vi "Server Main.vi"() -> ()   [LabVIEW 2024]
doc: "This VI is the main VI of the server."
uses:
  Controls/Server/Server - Data.ctl
  Support/Shared/Message Queue/Server Message Queues.ctl
  Support/Shared/Message Queue/Message Cluster.ctl
  Controls/Server/Server Status.ctl
  Error Handlers/Error Message.ctl
  Controls/Server/Historical Log.ctl
  Globals/Global - Server.vi
  Support/Shared/Message Queue.lvlib
  Support/Shared/User Event - Stop.lvlib
panel:
  in  "Exit":bool
  out "Status Log":i32(listbox)=-1
  in  "Administrator Console":bool
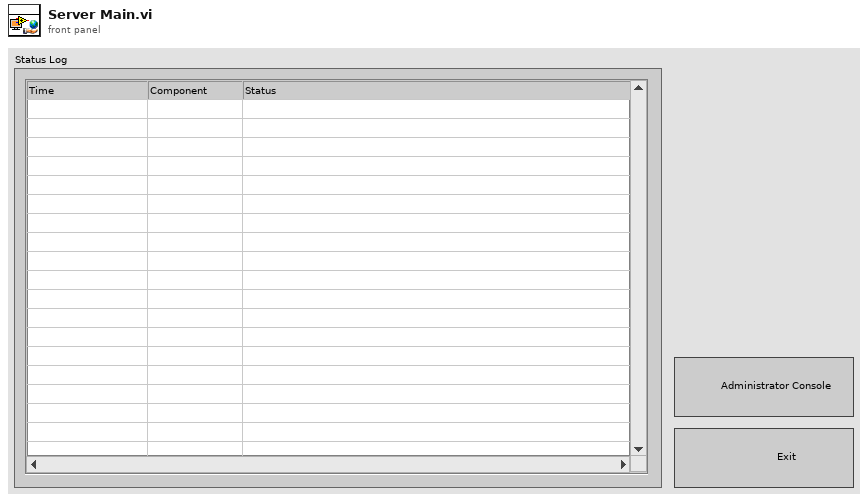
[diagram p1: front panel]
types:
  T1 = typedef "Server Status.ctl" = enum16{"Started", "Initialized", "Stopping", "Stopped"}
  T2 = typedef "Server - Data.ctl" = cluster{"UI Message Loop Initialized?":bool, "Shared Variable Management Loop Initialized?":bool, "Archive Loop Initialized?":bool, "Shared Variable Management Loop Stopped?":bool, "Archive Loop Stopped?":bool, "Administrator Console VI Reference":refnum<vi>, "Server Stop Handler":refnum<user-event>, "Server Message Queues":T3, "Server Status":T1, "Status Log Control":refnum<vi>}
  T3 = typedef "Message Queue.lvlib/Server Message Queues.ctl" = cluster{"UI":refnum<queue>, "Archive":refnum<queue>, "Shared Variable Management":refnum<queue>, "Administrator Console":refnum<queue>}
  T4 = typedef "Error Message.ctl" = cluster{"Error":errorcluster, "Component":string}
  T5 = typedef "Historical Log.ctl" = cluster{"Time":timestamp, "Component":string, "Status":string}
  T6 = typedef "System Configuration.ctl" = cluster{"Name":string, "Description":string, "Logging Computer Name":string, "Logging Database Name":string, "Logging Database Path":path, "Archive Computer Name":string, "Archive Database Name":string, "Archive Database Path":path, "Lifespan (days)":u32, "Archive Enabled":bool, "Archive Interval (hours)":u32, "Subsystems":T7[]}
  T7 = typedef "Subsystem Configuration.ctl" = cluster{"Name":string, "Root URL":refnum<k21>}
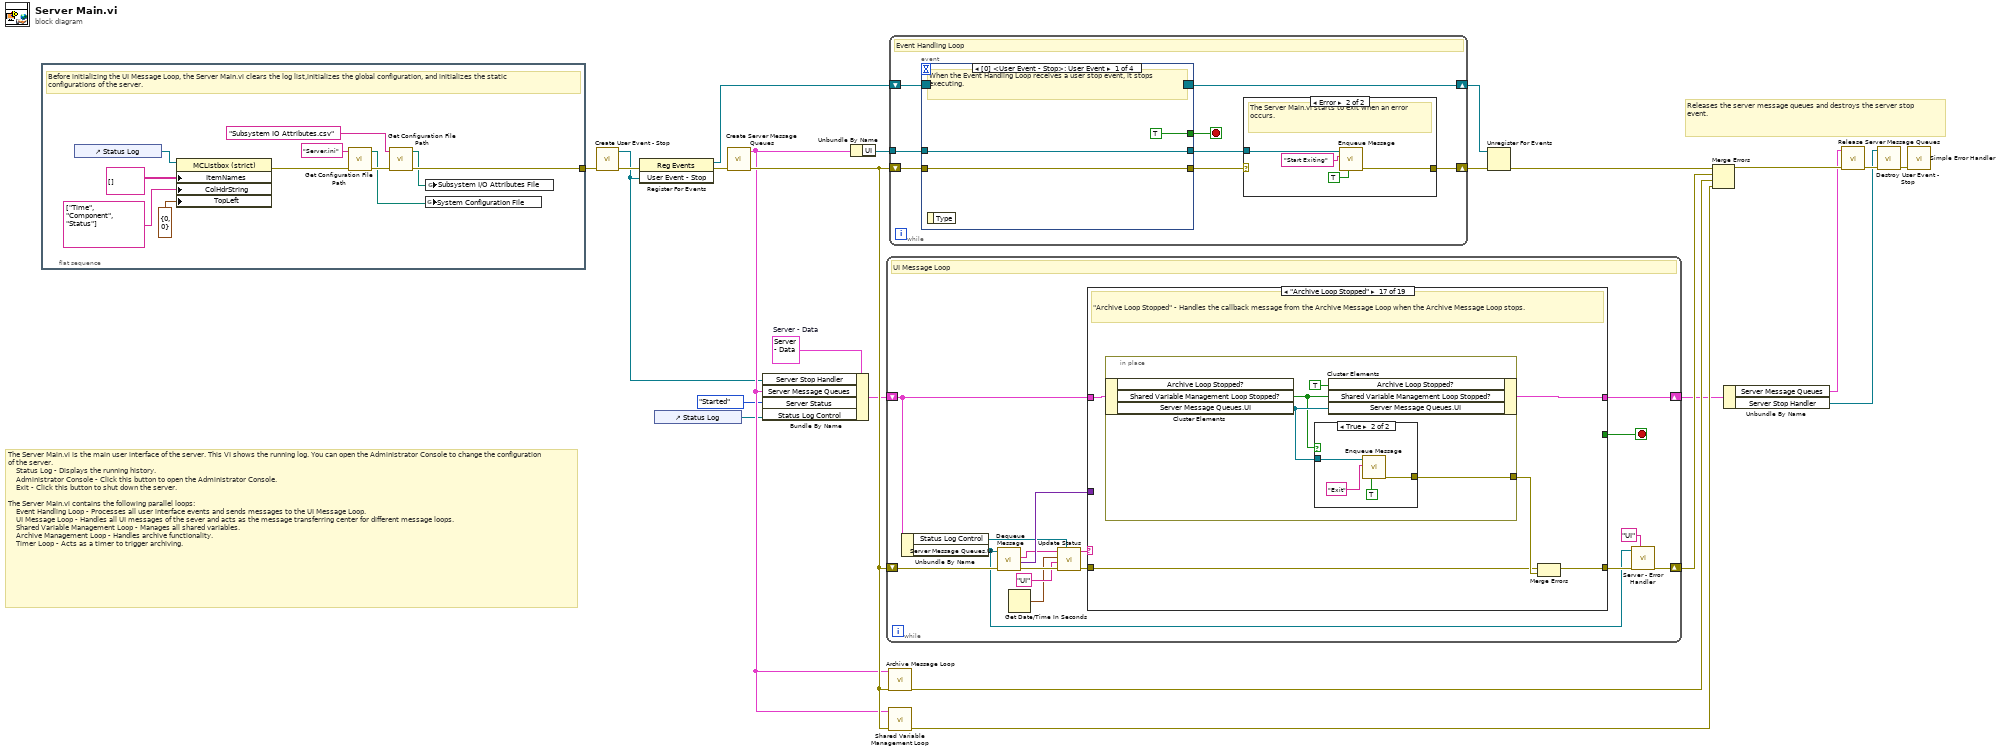
[diagram p0: block diagram]
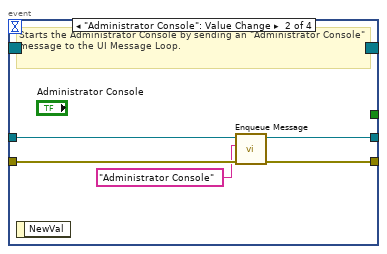
[diagram p3: hidden frame]
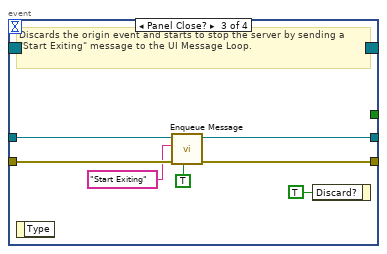
[diagram p4: hidden frame]
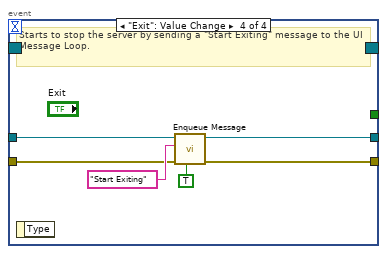
[diagram p5: hidden frame]
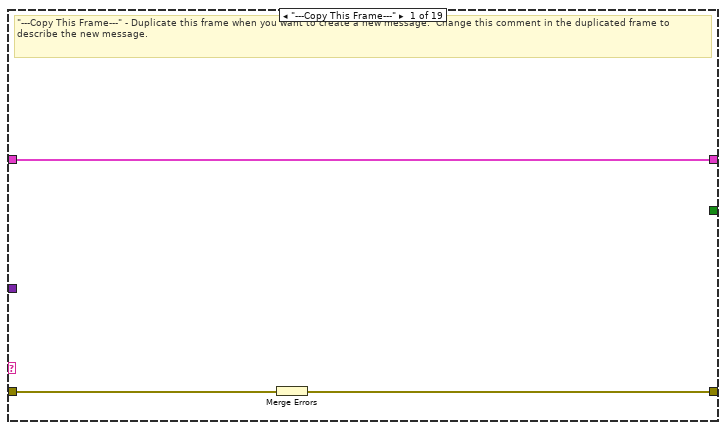
[diagram p6: hidden frame]
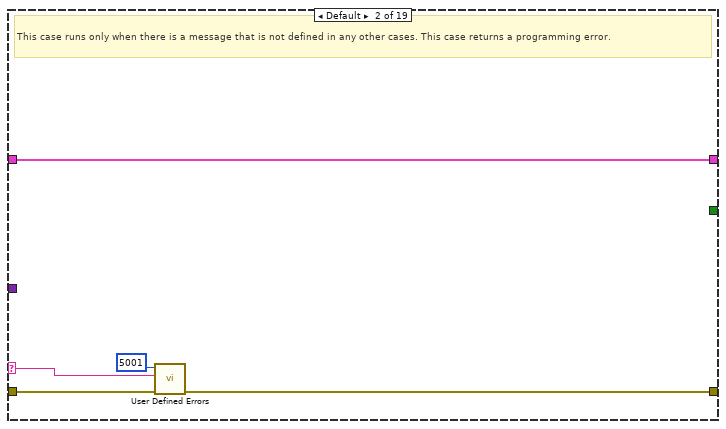
[diagram p7: hidden frame]
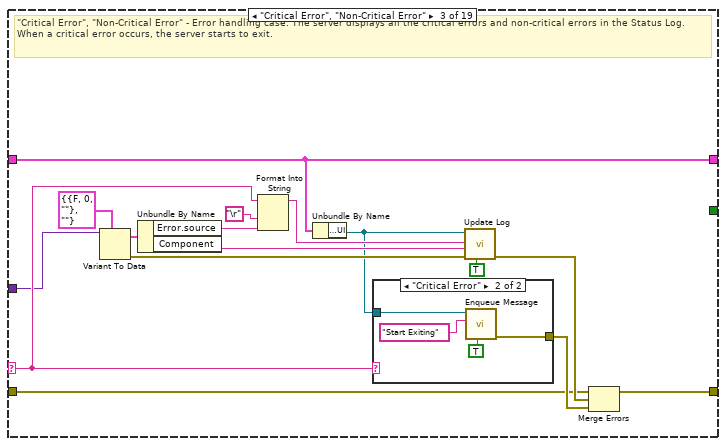
[diagram p8: hidden frame]
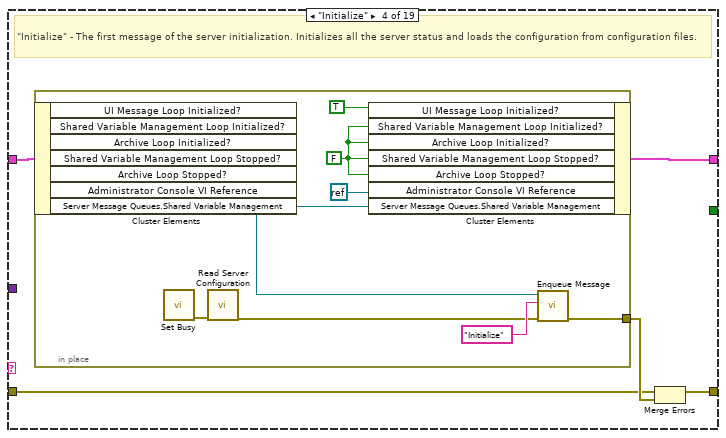
[diagram p10: hidden frame]
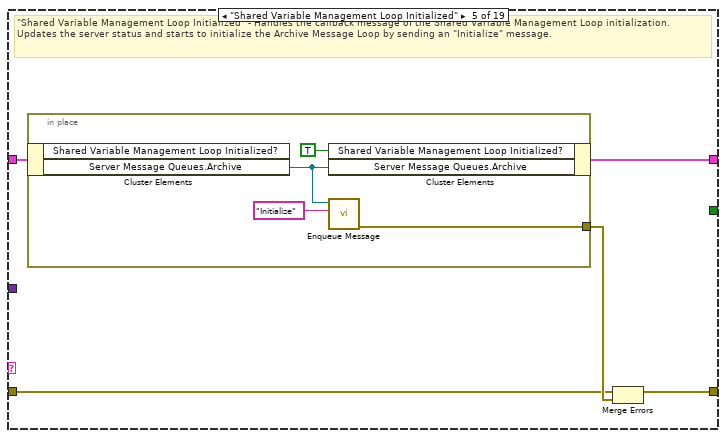
[diagram p11: hidden frame]
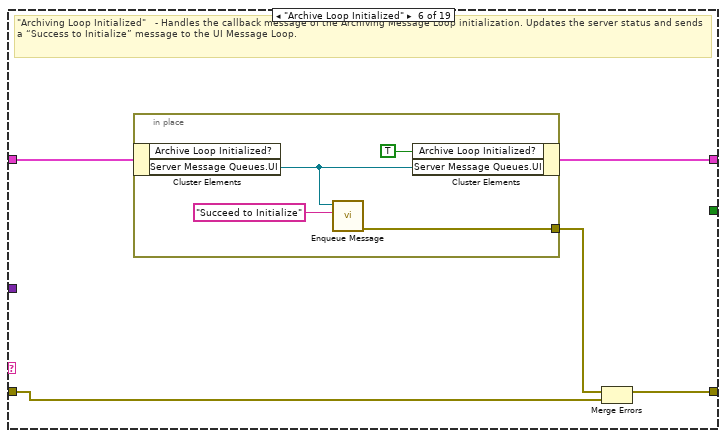
[diagram p12: hidden frame]
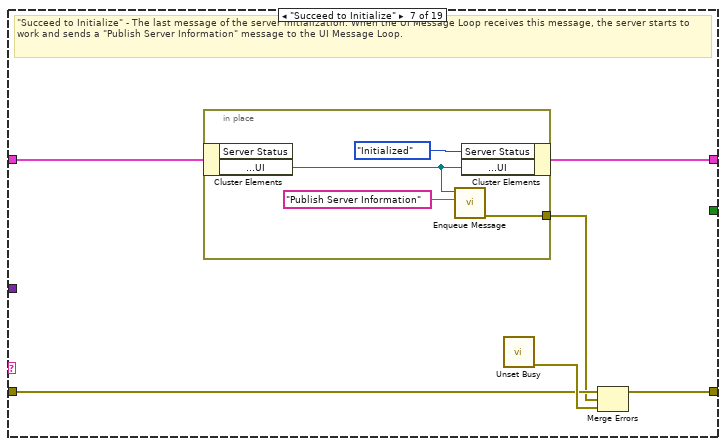
[diagram p13: hidden frame]
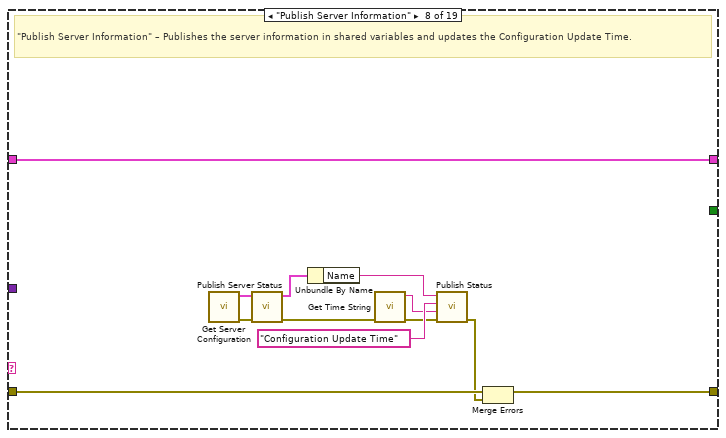
[diagram p14: hidden frame]
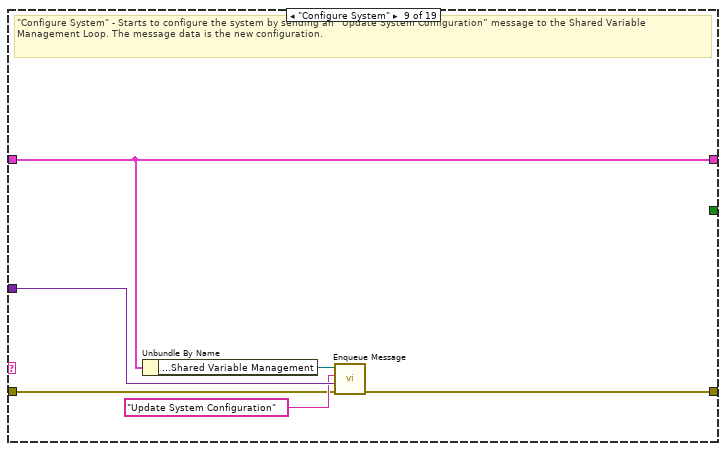
[diagram p15: hidden frame]
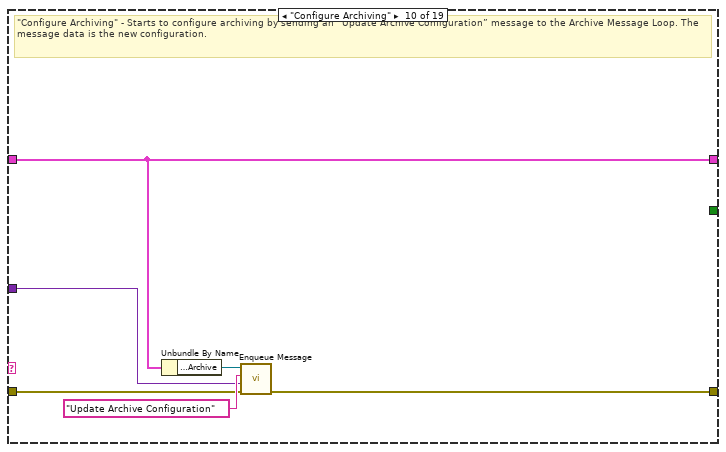
[diagram p16: hidden frame]
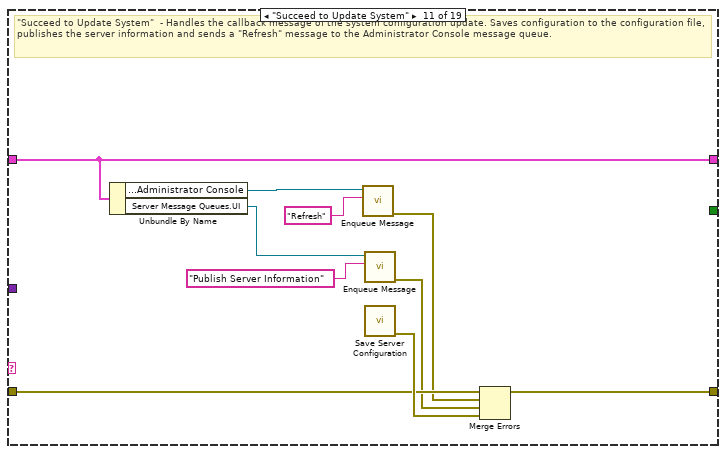
[diagram p17: hidden frame]
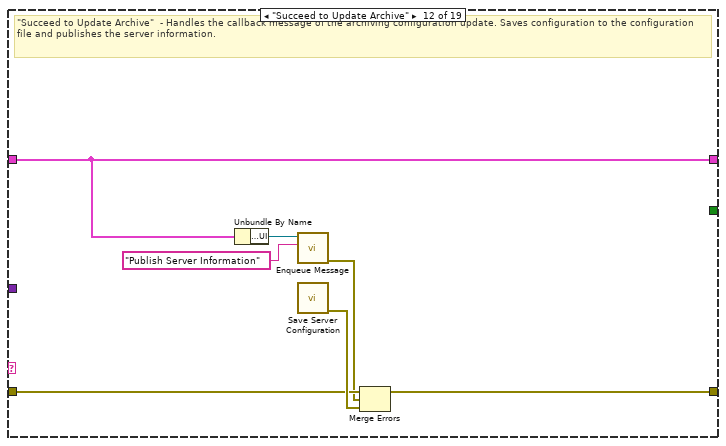
[diagram p18: hidden frame]
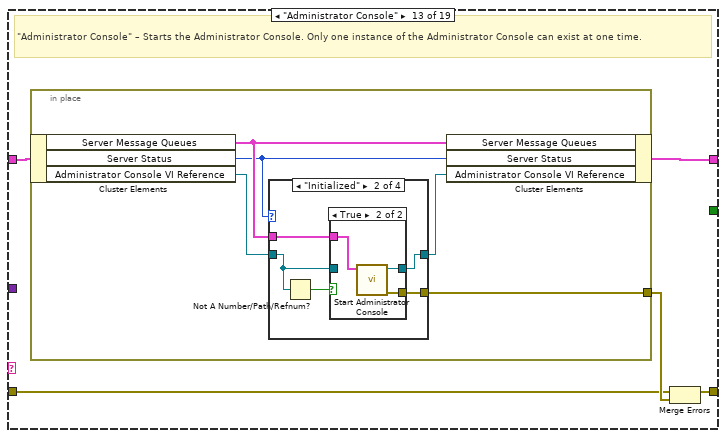
[diagram p19: hidden frame]
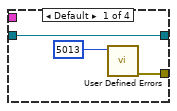
[diagram p20: hidden frame]
diagram:
  w12 = T2 {"UI Message Loop Initialized?"=FALSE, "Shared Variable Management Loop Initialized?"=FALSE, "Archive Loop Initialized?"=FALSE, "Shared Variable Management Loop Stopped?"=FALSE, "Archive Loop Stopped?"=FALSE, "Administrator Console VI Reference"=refnum, "Server Stop Handler"=refnum, "Server Message Queues"={"UI"=refnum, "Archive"=refnum, "Shared Variable Management"=refnum, "Administrator Console"=refnum}, "Server Status"=enum."Started", "Status Log Control"=refnum}  # Server - Data
  # "Releases the server message queues and destroys the server stop event."
  # "The Server Main.vi is the main user interface of the server. This VI shows the running log. You can open the Administrator Console to change the configuration of the server. \n    Status Log - Displays the running history.\n    Administrator Console - Click this button to open the Administrator Console.\n    Exit - Click this button to shut down the server.\n\nThe Server Main.vi contains the following parallel loops:\n    Event Handling Loop - Processes all user interface events and sends messages to the UI Message Loop.\n    UI Message Loop - Handles all UI messages of the sever and acts as the message transferring center for different message loops.\n    Shared Variable Management Loop - Manages all shared variables. \n    Archive Management Loop - Handles archive functionality.\n    Timer Loop - Acts as a timer to trigger archiving."
  n1 = flat-sequence {
    tunnel: [w28] -> w15
    frame #0 {
      # "Before initializing the UI Message Loop, the Server Main.vi clears the log list,initializes the global configuration, and initializes the static configurations of the server."
      n2 = control-ref of="Status Log"() -> (w33:refnum<vi>)
      n3 = property class="MCListbox (strict)"(reference=w33, "ItemNames"=string[][] [] ("Item Names"), "ColHdrString"=string[] ["Time", "Component", "Status"] ("Column Header Strings[]"), "TopLeft"=cluster{"Row":u32, "Column":u32} {"Row"=0, "Column"=0} ("Top Left Visible Cell")) -> (error out=w30:errorcluster)  [unwired: 1 in, 1 out]
      n4 = call "Get Configuration File Path.vi"("error in (no error)"=w30, "Configuration File Name"="Server.ini") -> ("error out"=w29:errorcluster, "Configuration File Path"=w26:path)  [unwired: 8 in]
      n5 = call "Get Configuration File Path.vi"("error in (no error)"=w29, "Configuration File Name"="Subsystem IO Attributes.csv") -> ("error out"=w28:errorcluster, "Configuration File Path"=w25:path)  [unwired: 8 in]
      n6 = global write "Global - Server.vi" "System Configuration File"(w26) -> ()
      n7 = global write "Global - Server.vi" "Subsystem I/O Attributes File"(w25) -> ()
    }
  }
  n8 = call "Create User Event - Stop.vi"("error in (no error)"=w15) -> ("error out"=w4:errorcluster, "User Event - Stop"=w1:refnum<user-event>)  [unwired: 9 in]
  n9 = register-events(error in=w4, w1) -> (reference out=w2:refnum<event-registration>, error out=w3:errorcluster)  [unwired: 1 in]
  n10 = control-ref of="Status Log"() -> (w5:refnum<vi>)
  n11 = call "Create Server Message Queues.vi"("error in (no error)"=w3) -> ("error out"=w17:errorcluster, "Message Queues Out"=w10:T3)  [unwired: 9 in]
  n12 = Bundle By Name(cluster=w12, "Server Stop Handler"=w1, "Server Message Queues"=w10, "Server Status"=Server_Status."Started", "Status Log Control"=w5) -> (w11:T2)
  n13 = Unbundle By Name(w10) -> ("UI"=w16:refnum<queue>)
  n14 = while "UI Message Loop" {
    shift-right: [w38] -> w9
    shift-left: w11 -> [w36]
    shift-right: [w43] -> w24
    shift-left: w17 -> [w51]
    stop <- w50 stop-if-true
    # "UI Message Loop"
    n15 = Unbundle By Name(w36) -> ("Status Log Control"=w37:refnum<vi>, "Server Message Queues.UI"=w40:refnum<queue>)
    n16 = call "Dequeue Message.vi"("error in (no error)"=w51, "Message Queue"=w40) -> ("error out"=w48:errorcluster, "Message Data"=w49:variant, "Message"=w46:string)  [unwired: 6 in, 1 out]
    n17 = Get Date/Time In Seconds() -> (seconds since 1Jan1904=w41:timestamp)
    n18 = call "Update Status.vi"("Status Listbox"=w37, "error in (no error)"=w48, "Component"="UI" ("Msg Queue"), "Time"=w41, "Status"=w46) -> ("error out"=w47:errorcluster, "dup Status"=w45:string)  [unwired: 5 in]
    n19 = case "Message Cases" shown="\"Archive Loop Stopped\"" w45 {
      selector: w45 -> [_ w56 w67 _ _ _ _ _ _ _ _ _ _ _ _ _ _ _ _]
      tunnel: w47 -> [w54 w55 w60 w80 w93 w102 w114 w131 w135 w139 w149 w159 w164 w194 w205 w224 w243 w256 w269]
      tunnel: [w53 w58 w65 w82 w95 w106 w116 w132 w133 w142 w154 w161 w165 w195 w206 w225 w245 w258 w272] -> w44
      tunnel: w36 -> [w52 w57 w68 w84 w97 w105 w113 w127 w134 w141 w153 w156 w163 w193 w208 w223 w247 w260 w278]
      tunnel: [_ _ _ _ _ _ _ _ _ _ _ _ _ _ _ _ _ _ TRUE] -> w50
      tunnel: w49 -> [_ _ w66 _ _ _ _ _ w138 w140 _ _ _ _ w215 _ _ _ _]
      tunnel: [w52 w57 w68 w83 w96 w104 w112 w127 w134 w141 w153 w156 w162 w192 w208 w218 w246 w259 w278] -> w38
      frame "---Copy This Frame---" {
        # "\"---Copy This Frame---\" - Duplicate this frame when you want to create a new message.  Change this comment in the duplicated frame to describe the new message."
        n20 = Merge Errors(w54) -> (w53:errorcluster)
      }
      frame Default {
        # "This case runs only when there is a message that is not defined in any other cases. This case returns a programming error."
        n21 = call "User Defined Errors.vi"("error in (no error)"=w55, "Parameter 1"=w56, "Error Code (0)"=5001 ("error code (0)")) -> ("error out"=w58:errorcluster)  [unwired: 8 in]
      }
      frame "Critical Error", "Non-Critical Error" {
        # "\"Critical Error\", \"Non-Critical Error\" - Error handling case. The server displays all the critical errors and non-critical errors in the Status Log. When a critical error occurs, the server starts to exit."
        n22 = Variant To Data(type=T4 {"Error"={"status"=FALSE, "code"=0, "source"=""}, "Component"=""} ("Error Message"), Variant=w66) -> (data=w75:T4, error out=w69:errorcluster)  [unwired: 1 in]
        n23 = Unbundle By Name(w75) -> ("Error.source"=w72:string, "Component"=w70:string)
        n24 = Format Into String(initial string=w67, "\r", w72) -> (resulting string=w71:string)  [unwired: 2 in, 1 out]
        n25 = Unbundle By Name(w68) -> ("Server Message Queues.UI"=w63:refnum<queue>)
        n26 = case shown="\"Critical Error\"" w67 {
          tunnel: w63 -> [_ w79]
          tunnel: [_ w76] -> w64
          frame Default {
          }
          frame "Critical Error" {
            n27 = call "Enqueue Message.vi"("Priority Message? (F)"=TRUE, "Message"="Start Exiting", "Message Queue"=w79) -> ("error out"=w76:errorcluster)  [unwired: 7 in, 1 out]
          }
        }
        n28 = call "Update Log.vi"("Priority Message? (F)"=TRUE, "error in (no error)"=w69, "Component"=w70, "Status"=w71, "UI Message Queue"=w63) -> ("error out"=w62:errorcluster)  [unwired: 4 in, 2 out]
        n29 = Merge Errors(w60, w62, w64) -> (w65:errorcluster)
      }
      frame "Initialize" {
        # "\"Initialize\" - The first message of the server initialization. Initializes all the server status and loads the configuration from configuration files."
        n30 = in-place {
          in-place-border: [w90] -> w81
          w87 = FALSE ("Administrator Console Opened?")
          n31 = in-place-cluster #1(w84) -> ("Server Message Queues.Shared Variable Management"=w88:refnum<queue>)  [unwired: 6 out]
          n32 = call <vilib>:"Set Busy.vi"() -> ("error out"=w86:errorcluster)  [unwired: 10 in, 1 out]
          n33 = call "Read Server Configuration.vi"("error in (no error)"=w86) -> ("error out"=w91:errorcluster)  [unwired: 10 in]
          n34 = in-place-cluster #1("UI Message Loop Initialized?"=TRUE, "Shared Variable Management Loop Initialized?"=w87, "Archive Loop Initialized?"=w87, "Shared Variable Management Loop Stopped?"=w87, "Archive Loop Stopped?"=w87, "Administrator Console VI Reference"=refnum<k0> refnum, "Server Message Queues.Shared Variable Management"=w88) -> (w83:T2)
          n35 = call "Enqueue Message.vi"("error in (no error)"=w91, "Message"="Initialize", "Message Queue"=w88) -> ("error out"=w90:errorcluster)  [unwired: 7 in, 1 out]
        }
        n36 = Merge Errors(w80, w81) -> (w82:errorcluster)
      }
      frame "Shared Variable Management Loop Initialized" {
        # "\"Shared Variable Management Loop Initialized\" - Handles the callback message of the Shared Variable Management Loop initialization. Updates the server status and starts to initialize the Archive Message Loop by sending an \"Initialize\" message."
        n37 = in-place {
          in-place-border: [w98] -> w94
          n38 = in-place-cluster #2(w97) -> ("Server Message Queues.Archive"=w99:refnum<queue>)  [unwired: 1 out]
          n39 = in-place-cluster #2("Shared Variable Management Loop Initialized?"=TRUE, "Server Message Queues.Archive"=w99) -> (w96:T2)
          n40 = call "Enqueue Message.vi"("Message"="Initialize", "Message Queue"=w99) -> ("error out"=w98:errorcluster)  [unwired: 8 in, 1 out]
        }
        n41 = Merge Errors(w93, w94) -> (w95:errorcluster)
      }
      frame "Archive Loop Initialized" {
        # "\"Archiving Loop Initialized\"   - Handles the callback message of the Archiving Message Loop initialization. Updates the server status and sends a “Success to Initialize” message to the UI Message Loop."
        n42 = in-place {
          in-place-border: [w107] -> w103
          n43 = in-place-cluster #3(w105) -> ("Server Message Queues.UI"=w108:refnum<queue>)  [unwired: 1 out]
          n44 = call "Enqueue Message.vi"("Message"="Succeed to Initialize", "Message Queue"=w108) -> ("error out"=w107:errorcluster)  [unwired: 8 in, 1 out]
          n45 = in-place-cluster #3("Archive Loop Initialized?"=TRUE, "Server Message Queues.UI"=w108) -> (w104:T2)
        }
        n46 = Merge Errors(w103, w102) -> (w106:errorcluster)
      }
      frame "Succeed to Initialize" {
        # "\"Succeed to Initialize\" - The last message of the server initialization. When the UI Message Loop receives this message, the server starts to work and sends a \"Publish Server Information\" message to the UI Message Loop."
        n47 = in-place {
          in-place-border: [w118] -> w111
          n48 = in-place-cluster #4(w113) -> ("Server Message Queues.UI"=w119:refnum<queue>)  [unwired: 1 out]
          n49 = call "Enqueue Message.vi"("Message"="Publish Server Information", "Message Queue"=w119) -> ("error out"=w118:errorcluster)  [unwired: 8 in, 1 out]
          n50 = in-place-cluster #4("Server Status"=Server_Status."Initialized", "Server Message Queues.UI"=w119) -> (w112:T2)
        }
        n51 = call <vilib>:"Unset Busy.vi"() -> ("error out"=w115:errorcluster)  [unwired: 11 in]
        n52 = Merge Errors(w114, w111, w115) -> (w116:errorcluster)
      }
      frame "Publish Server Information" {
        # "\"Publish Server Information\" – Publishes the server information in shared variables and updates the Configuration Update Time."
        n53 = call "Get Server Configuration.vi"() -> ("error out"=w124:errorcluster, "System Configuration"=w126:T6)  [unwired: 9 in, 1 out]
        n54 = call "Publish Server Status.vi"("error in (no error)"=w124, "System Configuration"=w126) -> ("error out"=w123:errorcluster, "dup System Configuration"=w125:T6)  [unwired: 8 in]
        n55 = Unbundle By Name(w125) -> ("Name"=w128:string)
        n56 = call "Get Time String.vi"("error in (no error)"=w123) -> ("error out"=w122:errorcluster, "Time String"=w121:string)  [unwired: 9 in]
        n57 = call "Publish Status.vi"("error in (no error)"=w122, "Value"=w121, "Parameter"="Configuration Update Time", "System Name"=w128) -> ("error out"=w129:errorcluster)  [unwired: 7 in]
        n58 = Merge Errors(w131, w129) -> (w132:errorcluster)
      }
      frame "Configure System" {
        # "\"Configure System\" - Starts to configure the system by sending an “Update System Configuration” message to the Shared Variable Management Loop. The message data is the new configuration."
        n59 = Unbundle By Name(w134) -> ("Server Message Queues.Shared Variable Management"=w136:refnum<queue>)
        n60 = call "Enqueue Message.vi"("error in (no error)"=w135, "Message Data"=w138, "Message"="Update System Configuration", "Message Queue"=w136) -> ("error out"=w133:errorcluster)  [unwired: 6 in, 1 out]
      }
      frame "Configure Archiving" {
        # "\"Configure Archiving\" - Starts to configure archiving by sending an “Update Archive Configuration” message to the Archive Message Loop. The message data is the new configuration."
        n61 = Unbundle By Name(w141) -> ("Server Message Queues.Archive"=w144:refnum<queue>)
        n62 = call "Enqueue Message.vi"("error in (no error)"=w139, "Message Data"=w140, "Message"="Update Archive Configuration", "Message Queue"=w144) -> ("error out"=w142:errorcluster)  [unwired: 6 in, 1 out]
      }
      frame "Succeed to Update System" {
        # "\"Succeed to Update System\"  - Handles the callback message of the system configuration update. Saves configuration to the configuration file, publishes the server information and sends a \"Refresh\" message to the Administrator Console message queue."
        n63 = Unbundle By Name(w153) -> ("Server Message Queues.Administrator Console"=w152:refnum<queue>, "Server Message Queues.UI"=w145:refnum<queue>)
        n64 = call "Enqueue Message.vi"("Message"="Refresh", "Message Queue"=w152) -> ("error out"=w148:errorcluster)  [unwired: 8 in, 1 out]
        n65 = call "Enqueue Message.vi"("Message"="Publish Server Information", "Message Queue"=w145) -> ("error out"=w146:errorcluster)  [unwired: 8 in, 1 out]
        n66 = call "Save Server Configuration.vi"() -> ("error out"=w150:errorcluster)  [unwired: 11 in]
        n67 = Merge Errors(w149, w148, w146, w150) -> (w154:errorcluster)
      }
      frame "Succeed to Update Archive" {
        # "\"Succeed to Update Archive\"  - Handles the callback message of the archiving configuration update. Saves configuration to the configuration file and publishes the server information."
        n68 = Unbundle By Name(w156) -> ("Server Message Queues.UI"=w157:refnum<queue>)
        n69 = call "Enqueue Message.vi"("Message"="Publish Server Information", "Message Queue"=w157) -> ("error out"=w155:errorcluster)  [unwired: 8 in, 1 out]
        n70 = call "Save Server Configuration.vi"() -> ("error out"=w160:errorcluster)  [unwired: 11 in]
        n71 = Merge Errors(w159, w155, w160) -> (w161:errorcluster)
      }
      frame "Administrator Console" {
        # "\"Administrator Console\" – Starts the Administrator Console. Only one instance of the Administrator Console can exist at one time."
        n72 = in-place {
          in-place-border: [w171] -> w166
          n73 = in-place-cluster #5(w163) -> ("Server Message Queues"=w170:T3, "Server Status"=w167:T1, "Administrator Console VI Reference"=w168:refnum<vi>)
          n74 = case shown="\"Initialized\"" w167 {
            tunnel: [w173 w179 w187 w190] -> w171
            tunnel: w170 -> [_ w178 _ _]
            tunnel: w168 -> [w172 w176 w186 w189]
            tunnel: [w172 w177 w186 w189] -> w169
            frame Default {
              n75 = call "User Defined Errors.vi"("Error Code (0)"=5013 ("error code (0)")) -> ("error out"=w173:errorcluster)  [unwired: 10 in]
            }
            frame "Initialized" {
              n76 = Not A Number/Path/Refnum?(number/path/refnum=w176) -> (NaN/Path/Refnum?=w175:bool)
              n77 = case shown="True" w175 {
                tunnel: w176 -> [w182 _]
                tunnel: w178 -> [_ w184]
                tunnel: [w181 w185] -> w179
                tunnel: [w180 w183] -> w177
                frame False {
                  n78 = call "Bring VI to Topmost.vi"("VI Reference In"=w182) -> ("error out"=w181:errorcluster, "VI Reference Out"=w180:refnum<vi>)  [unwired: 9 in]
                }
                frame True {
                  n79 = call "Start Administrator Console.vi"("Message Queues"=w184) -> ("error out"=w185:errorcluster, "Administrator Console Reference"=w183:refnum<vi>)  [unwired: 9 in]
                }
              }
            }
            frame "Stopping" {
              n80 = call "User Defined Errors.vi"("Error Code (0)"=5015 ("error code (0)")) -> ("error out"=w187:errorcluster)  [unwired: 10 in]
            }
            frame "Started" {
              n81 = call "User Defined Errors.vi"("Error Code (0)"=5014 ("error code (0)")) -> ("error out"=w190:errorcluster)  [unwired: 10 in]
            }
          }
          n82 = in-place-cluster #5("Server Message Queues"=w170, "Server Status"=w167, "Administrator Console VI Reference"=w169) -> (w162:T2)
        }
        n83 = Merge Errors(w164, w166) -> (w165:errorcluster)
      }
      frame "Administrator Console Closed" {
        # "\"Administrator Console Closed\" - Handles the callback message from the Administrator Console when the Administrator Console is closed. Clears the saved Administrator Console VI reference."
        n84 = in-place {
          in-place-border: [w200] -> w196
          n85 = in-place-cluster #6(w193) -> ("Administrator Console VI Reference"=w197:refnum<vi>)
          n86 = Not A Number/Path/Refnum?(number/path/refnum=w197) -> (NaN/Path/Refnum?=w198:bool)
          n87 = case shown="False" w198 {
            tunnel: w197 -> [w202 w204]
            tunnel: [w203 _] -> w200
            tunnel: [refnum<k0> refnum w204] -> w199
            frame False {
              n88 = Close Reference(reference=w202) -> (error out=w203:errorcluster)  [unwired: 1 in]
            }
            frame True {
            }
          }
          n89 = in-place-cluster #6("Administrator Console VI Reference"=w199) -> (w192:T2)
        }
        n90 = Merge Errors(w194, w196) -> (w195:errorcluster)
      }
      frame "Update Display" {
        # "\"Update Display\" – Updates the Status Log."
        n91 = Variant To Data(type=T5 {"Time"=timestamp(0 s since 1904-01-01), "Component"="", "Status"=""} ("log"), Variant=w215) -> (data=w213:T5, error out=w216:errorcluster)  [unwired: 1 in]
        n92 = Unbundle By Name(w208) -> ("Status Log Control"=w207:refnum<vi>)
        n93 = Unbundle By Name(w213) -> ("Status"=w210:string, "Time"=w211:timestamp, "Component"=w212:string)
        n94 = call "Update Status.vi"("Status Listbox"=w207, "error in (no error)"=w216, "Component"=w212, "Time"=w211, "Status"=w210) -> ("error out"=w209:errorcluster)  [unwired: 5 in, 1 out]
        n95 = Merge Errors(w205, w209) -> (w206:errorcluster)
      }
      frame "Start Exiting" {
        # "\"Start Exiting\"  - The first message of stopping the server. Changes the server status, starts to stop the Administrator Console, the Archive Message Loop and the Shared Variable Management Loop by sending “Exit” messages."
        n96 = Unbundle By Name(w223) -> ("Server Message Queues.Shared Variable Management"=w222:refnum<queue>, "Server Message Queues.Archive"=w221:refnum<queue>, "Server Message Queues.Administrator Console"=w220:refnum<queue>, "Server Status"=w219:T1)
        n97 = call <vilib>:"Set Busy.vi"() -> ("error out"=w217:errorcluster)  [unwired: 10 in, 1 out]
        n98 = case shown="Default" w219 {
          tunnel: [w238 w241] -> w225
          tunnel: w224 -> [w227 w240]
          tunnel: w223 -> [w231 w239]
          tunnel: w222 -> [w234 _]
          tunnel: w221 -> [w233 _]
          tunnel: w220 -> [w232 _]
          tunnel: [w229 w239] -> w218
          tunnel: w217 -> [w226 _]
          frame Default {
            w228 = "Exit" ("Message")
            n99 = call "Enqueue Message.vi"("error in (no error)"=w226, "Message"=w228, "Message Queue"=w234) -> ("error out"=w237:errorcluster)  [unwired: 7 in, 1 out]
            n100 = call "Enqueue Message.vi"("error in (no error)"=w226, "Message"=w228, "Message Queue"=w233) -> ("error out"=w236:errorcluster)  [unwired: 7 in, 1 out]
            n101 = call "Enqueue Message.vi"("error in (no error)"=w226, "Message"=w228, "Message Queue"=w232) -> ("error out"=w235:errorcluster)  [unwired: 7 in, 1 out]
            n102 = Bundle By Name(cluster=w231, "Server Status"=Server_Status."Stopping") -> (w229:T2)
            n103 = Merge Errors(w227, w237, w236, w235) -> (w238:errorcluster)
          }
          frame "Stopping" {
            n104 = call "User Defined Errors.vi"("error in (no error)"=w240, "Error Code (0)"=5012 ("error code (0)")) -> ("error out"=w241:errorcluster)  [unwired: 9 in]
          }
        }
      }
      frame "Archive Loop Stopped" {
        # "\"Archive Loop Stopped\" - Handles the callback message from the Archive Message Loop when the Archive Message Loop stops."
        n105 = in-place {
          in-place-border: [w248] -> w244
          n106 = in-place-cluster #7(w247) -> ("Shared Variable Management Loop Stopped?"=w249:bool, "Server Message Queues.UI"=w250:refnum<queue>)  [unwired: 1 out]
          n107 = case shown="True" w249 {
            tunnel: [_ w253] -> w248
            tunnel: w250 -> [_ w252]
            frame False {
            }
            frame True {
              n108 = call "Enqueue Message.vi"("Priority Message? (F)"=TRUE, "Message"="Exit", "Message Queue"=w252) -> ("error out"=w253:errorcluster)  [unwired: 7 in, 1 out]
            }
          }
          n109 = in-place-cluster #7("Archive Loop Stopped?"=TRUE, "Shared Variable Management Loop Stopped?"=w249, "Server Message Queues.UI"=w250) -> (w246:T2)
        }
        n110 = Merge Errors(w243, w244) -> (w245:errorcluster)
      }
      frame "Shared Variable Management Loop Stopped" {
        # "\"Shared Variable Management Loop Stopped\" -  Handles the callback message from the Shared Variable Management Loop when the Shared Variable Management Loop stops."
        n111 = in-place {
          in-place-border: [w261] -> w257
          n112 = in-place-cluster #8(w260) -> ("Archive Loop Stopped?"=w262:bool, "Server Message Queues.UI"=w263:refnum<queue>)  [unwired: 1 out]
          n113 = case shown="True" w262 {
            tunnel: [_ w266] -> w261
            tunnel: w263 -> [_ w265]
            frame False {
            }
            frame True {
              n114 = call "Enqueue Message.vi"("Priority Message? (F)"=TRUE, "Message"="Exit", "Message Queue"=w265) -> ("error out"=w266:errorcluster)  [unwired: 7 in, 1 out]
            }
          }
          n115 = in-place-cluster #8("Shared Variable Management Loop Stopped?"=TRUE, "Archive Loop Stopped?"=w262, "Server Message Queues.UI"=w263) -> (w259:T2)
        }
        n116 = Merge Errors(w256, w257) -> (w258:errorcluster)
      }
      frame "Exit" {
        # "#CodeNeeded - Clear your own allocated resource."
        # "\"Exit\" – When the UI Message Loop receives this message, it stops. Clears data and stops the Event Handling Loop by triggering the server stop event."
        n117 = global read "Global - Server.vi" "Subsystem I/O Attributes"() -> (w275:refnum<data-value>)
        n118 = global read "Global - Server.vi" "System Configuration"() -> (w276:refnum<data-value>)
        n119 = Unbundle By Name(w278) -> ("Server Stop Handler"=w277:refnum<user-event>)
        n120 = call "Fire User Event - Stop.vi"("User Event - Stop"=w277) -> ("error out"=w279:errorcluster)  [unwired: 10 in]
        n121 = Delete Data Value Reference(data value reference=w276) -> (error out=w273:errorcluster)  [unwired: 1 in, 1 out]
        n122 = Delete Data Value Reference(data value reference=w275) -> (error out=w274:errorcluster)  [unwired: 1 in, 1 out]
        n123 = Merge Errors(w273, w274, w279) -> (w271:errorcluster)
        n124 = call <vilib>:"Unset Busy.vi"("error in (no error)"=w271) -> ("error out"=w270:errorcluster)  [unwired: 10 in]
        n125 = Merge Errors(w269, w270) -> (w272:errorcluster)
      }
    }
    n126 = call "Server - Error Handler.vi"("Component"="UI", "error in (no error)"=w44, "Message Queue"=w40) -> ("error out"=w43:errorcluster)  [unwired: 8 in]
  }
  n127 = call "Archive Message Loop.vi"("error in (no error)"=w17, "Message Queues"=w10) -> ("error out"=w20:errorcluster)  [unwired: 9 in]
  n128 = call "Shared Variable Management Loop.vi"("error in (no error)"=w17, "Message Queues"=w10) -> ("error out"=w19:errorcluster)  [unwired: 9 in]
  n129 = while "Event Handling Loop" {
    tunnel: w16 -> [w284]
    shift-right: [w286] -> w18
    shift-left: w2 -> [w287]
    shift-right: [w281] -> w21
    shift-left: w17 -> [w288]
    stop <- w285 stop-if-true
    # "Event Handling Loop"
    n130 = event shown="[0] <User Event - Stop>: User Event" {
      selector: w287 -> [_ _ _ _]
      dyn-events: [_ _ _ _] -> w286
      timeout: _ -> [_ _ _ _]
      tunnel: [TRUE ("Discard?") _ _ _] -> w285
      tunnel: w284 -> [w294 w301 w307 w312]
      tunnel: [w296 w300 w306 w309] -> w283
      tunnel: w288 -> [w296 w299 w304 w310]
      tunnel: [w294 w297 w303 w311] -> w282
      event User Event {
        # "When the Event Handling Loop receives a user stop event, it stops executing."
        n131 = event-data() -> ()  [unwired: 1 in, 1 out]
      }
      event "Administrator Console": Value Change {
        # "Starts the Administrator Console by sending an \"Administrator Console\" message to the UI Message Loop."
        n132 = event-data() -> ()  [unwired: 1 in, 1 out]
        n133 = call "Enqueue Message.vi"("error in (no error)"=w299, "Message"="Administrator Console", "Message Queue"=w301) -> ("error out"=w300:errorcluster, "dup Message Queue"=w297:refnum<queue>)  [unwired: 7 in]
      }
      event Panel Close? {
        # "Discards the origin event and starts to stop the server by sending a \"Start Exiting\" message to the UI Message Loop."
        n134 = event-data() -> ()  [unwired: 1 in, 1 out]
        n135 = call "Enqueue Message.vi"("Priority Message? (F)"=TRUE, "error in (no error)"=w304, "Message"="Start Exiting", "Message Queue"=w307) -> ("error out"=w306:errorcluster, "dup Message Queue"=w303:refnum<queue>)  [unwired: 6 in]
        n136 = event-data("Discard?"=TRUE) -> ()  [unwired: 1 in, 1 out]
      }
      event "Exit": Value Change {
        # "Starts to stop the server by sending a \"Start Exiting\" message to the UI Message Loop."
        n137 = event-data() -> ()  [unwired: 1 in, 1 out]
        n138 = call "Enqueue Message.vi"("Priority Message? (F)"=TRUE, "error in (no error)"=w310, "Message"="Start Exiting", "Message Queue"=w312) -> ("error out"=w309:errorcluster, "dup Message Queue"=w311:refnum<queue>)  [unwired: 6 in]
      }
    }
    n139 = case "Event Handling Loop Error Handling" shown="Error" w283 {
      selector: w283 -> [w289 _]
      tunnel: w282 -> [_ w291]
      tunnel: [w289 w290] -> w281
      frame No Error {
        # "The Server Main.vi does nothing when no error occurs."
      }
      frame Error {
        # "The Server Main.vi starts to exit when an error occurs."
        n140 = call "Enqueue Message.vi"("Priority Message? (F)"=TRUE, "Message"="Start Exiting", "Message Queue"=w291) -> ("error out"=w290:errorcluster)  [unwired: 7 in, 1 out]
      }
    }
  }
  n141 = Unregister For Events(event registration refnum=w18, error in=w21) -> (error out=w22:errorcluster)
  n142 = Merge Errors(w22, w24, w20, w19) -> (w13:errorcluster)
  n143 = Unbundle By Name(w9) -> ("Server Message Queues"=w8:T3, "Server Stop Handler"=w7:refnum<user-event>)
  n144 = call "Release Server Message Queues.vi"("error in (no error)"=w13, "Server Message Queues"=w8) -> ("error out"=w14:errorcluster)  [unwired: 9 in]
  n145 = call "Destroy User Event - Stop.vi"("error in (no error)"=w14, "User Event - Stop"=w7) -> ("error out"=w23:errorcluster)  [unwired: 9 in]
  n146 = call <vilib>:"Simple Error Handler.vi"("error in (no error)"=w23) -> ()  [unwired: 4 in, 5 out]
